vi "Database.Init.vi"(8 "error in (no error)":errorcluster) -> (0 "error out":errorcluster)   [LabVIEW 2016]
uses:
  Database.Global.vi
  Database.Main.Data.Status.ctl
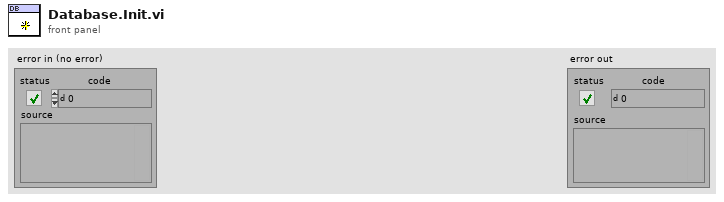
[diagram p1: front panel]
types:
  T1 = typedef "Database.Main.Data.Status.ctl" = cluster{"Run":bool, "Handle":i32, "ConnTS":timestamp, "DbTime":timestamp, "DbTimeCode":dbl, "DbTimeOffset":dbl}
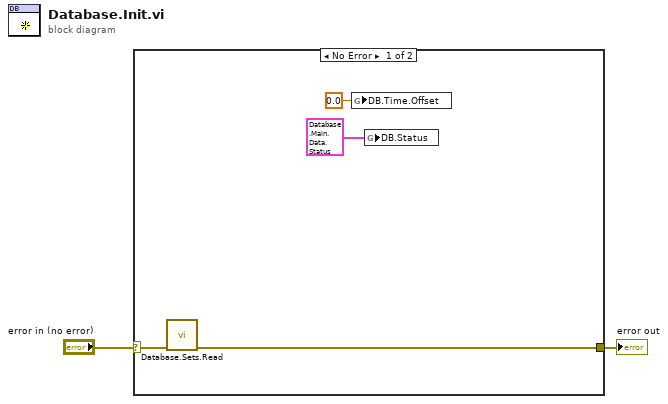
[diagram p0: block diagram]
diagram:
  n1 = case shown="No Error" "error in (no error)" {
    selector: "error in (no error)" -> [w6 w7]
    tunnel: [w3 w7] -> w1
    frame No Error {
      n2 = call "Database.Sets.Read.vi"("error in"=w6) -> ("error out"=w3:errorcluster)  [unwired: 10 in]
      n3 = global write "Database.Global.vi" "DB.Time.Offset"(0.0 ("DB.Time.Offset")) -> ()
      n4 = global write "Database.Global.vi" "DB.Status"(T1 {"Run"=FALSE, "Handle"=0, "ConnTS"=timestamp(0 s since 1904-01-01), "DbTime"=timestamp(0 s since 1904-01-01), "DbTimeCode"=0.0, "DbTimeOffset"=0.0} ("DB.Status")) -> ()
    }
    frame Error {
    }
  }
  "error out" <- w1
